vi "trig out logic.vi"(8 "rising edge":bool, 9 "Output Valid":bool, 10 "pulse idx":u8, 11 "state in":u16) -> (1 "output":bool, 3 "state out out":u16)   [LabVIEW 2018, in "trigger-out.lvlib"]
uses:
  trigger-out.lvlib
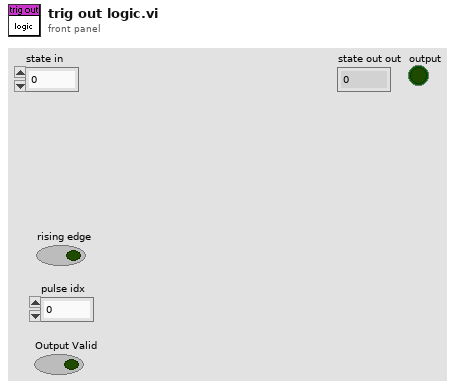
[diagram p1: front panel]
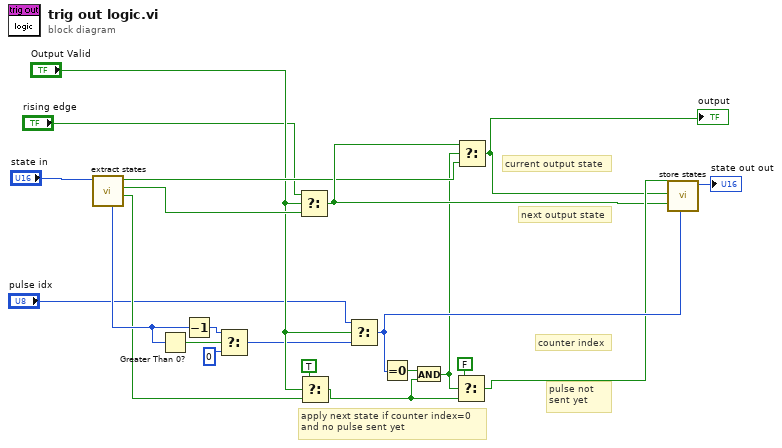
[diagram p0: block diagram]
diagram:
  # "apply next state if counter index=0 \nand no pulse sent yet"
  # "current output state"
  # "next output state"
  # "counter index"
  # "pulse not sent yet"
  n1 = call "extract states.vi"("state"="state in") -> ("pulse not yet sent"=w17:bool, "next output"=w16:bool, "current output"=w15:bool, "counter index"=w18:u8)  [unwired: 7 in]
  n2 = Greater Than 0?(x=w18) -> (x > 0?=w7:bool)
  n3 = Decrement(x=w18) -> (x-1=w8:u8)
  n4 = Select(t=w8, s=w7, f=u8 0) -> (s? t:f=w10:u8)
  n5 = Select(t="rising edge", s="Output Valid", f=w16) -> (s? t:f=w20:bool)
  n6 = Select(t=TRUE, s="Output Valid", f=w17) -> (s? t:f=w11:bool)
  n7 = Select(t="pulse idx", s="Output Valid", f=w10) -> (s? t:f=w22:u8)
  n8 = Equal To 0?(x=w22) -> (x = 0?=w12:bool)
  n9 = And(x=w12, y=w11) -> (x .and. y?=w13:bool)
  n10 = Select(t=FALSE, s=w13, f=w11) -> (s? t:f=w21:bool)
  n11 = Select(t=w20, s=w13, f=w15) -> (s? t:f=w19:bool)
  "output" <- w19
  n12 = call "store states.vi"("counter index"=w22, "pulse not yet sent"=w21, "next output"=w20, "current output"=w19) -> ("state out"=→"state out out":u16)  [unwired: 7 in]
